vi "3.1-Make XY Graph.vi"() -> (0 "3.1-Midbrain Arbitrated Graph":T1)   [LabVIEW 2010]
uses:
  3.1-Midbrain Arbitrated Graph.ctl
  4-High Neurons/4.1-Midbrain Act Data.ctl
  3.0-Global.vi
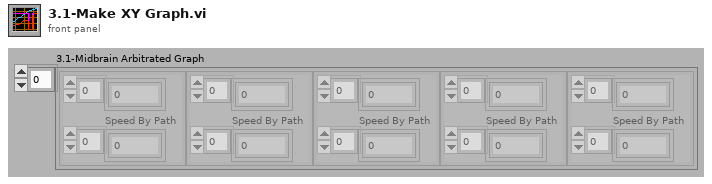
[diagram p1: front panel]
types:
  T1 = typedef "3.1-Midbrain Arbitrated Graph.ctl" = cluster{dbl[], "Speed By Path":dbl[]}[]
  T2 = enum16{"Set Joystick", "Read Joystick", "Set Forebrain", "Read Forebrain", "Set Limbic", "Read Limbic", "Set Cerebellum", "Read Cerebellum", "Set Arbitrated", "Read Arbitrated", "Set LIDAR", "Read LIDAR", "Read Shallow Map", "Set Shallow Map", "Read Decider", "Set Decider"}
  T3 = enum16{"Set Joystick", "Read Joystick", "Set Forebrain", "Read Forebrain", "Set Limbic", "Read Limbic", "Set Cerebellum", "Read Cerebellum", "Set Arbitrated", "Read Arbitrated", "Set LIDAR", "Read LIDAR", "Read Shallow Map", "Set Shallow Map"}
  T4 = enum16{"Set Midbrain Act Data", "Read Midbrain Act Data"}
  T5 = typedef "4.1-Midbrain Act Data.ctl" = cluster{"Arbitrated Array":sgl[], "Exploded Obstacles":sgl[], "Desired Change in Heading":sgl, "Desired Speed Fraction":sgl}
  T6 = enum16{"Steering Setpoints", "Desired Change in Heading"}
  T7 = enum16{"Set Joystick", "Read Joystick", "Set Forebrain", "Read Forebrain", "Set Limbic", "Read Limbic", "Set Cerebellum", "Read Cerebellum", "Set Arbitrated", "Read Arbitrated", "Set LIDAR", "Read LIDAR"}
  T8 = typedef "4.1.2-Act Neuron TD.ctl" = cluster{"Speed By Path":sgl[]}
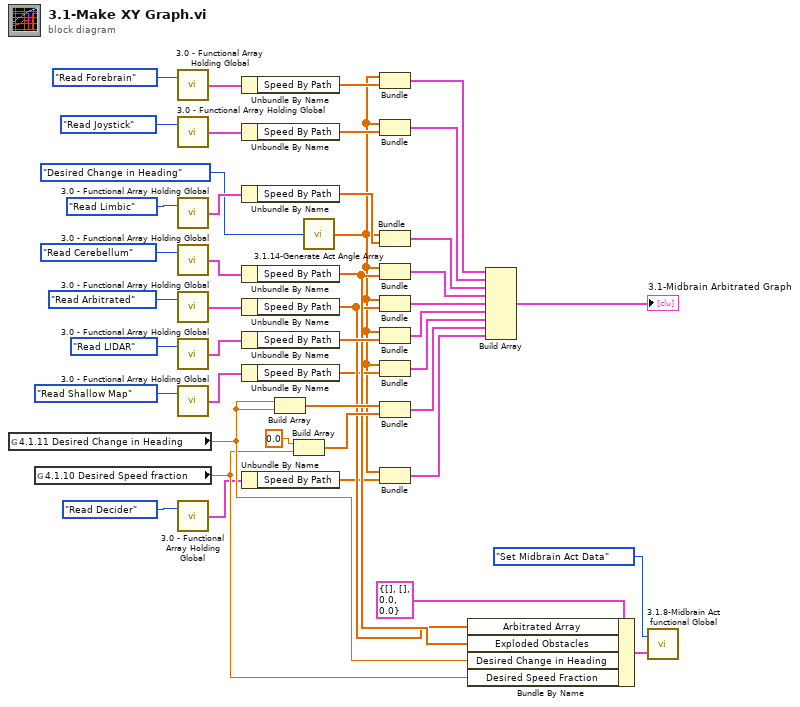
[diagram p0: block diagram]
diagram:
  n1 = global read "3.0-Global.vi" "4.1.11 Desired Change in Heading"() -> (w16:dbl)
  n2 = global read "3.0-Global.vi" "4.1.10 Desired Speed fraction"() -> (w11:dbl)
  n3 = call "3.0 - Functional Array Holding Global.vi"("Mode"=T7."Read Forebrain") -> ("Output Act Neurons"=w37:T8)  [unwired: 1 in]
  n4 = call "3.0 - Functional Array Holding Global.vi"("Mode"=T7."Read Joystick") -> ("Output Act Neurons"=w35:T8)  [unwired: 1 in]
  n5 = call "3.0 - Functional Array Holding Global.vi"("Mode"=T7."Read Limbic") -> ("Output Act Neurons"=w33:T8)  [unwired: 1 in]
  n6 = call "3.0 - Functional Array Holding Global.vi"("Mode"=T7."Read Cerebellum") -> ("Output Act Neurons"=w31:T8)  [unwired: 1 in]
  n7 = call "3.0 - Functional Array Holding Global.vi"("Mode"=T7."Read Arbitrated") -> ("Output Act Neurons"=w26:T8)  [unwired: 1 in]
  n8 = call "3.0 - Functional Array Holding Global.vi"("Mode"=T7."Read LIDAR") -> ("Output Act Neurons"=w29:T8)  [unwired: 1 in]
  n9 = call "3.0 - Functional Array Holding Global.vi"("Mode"=T3."Read Shallow Map") -> ("Output Act Neurons"=w9:T8)  [unwired: 1 in]
  n10 = call "3.0 - Functional Array Holding Global.vi"("Mode"=T2."Read Decider") -> ("Output Act Neurons"=w5:T8)  [unwired: 1 in]
  n11 = Unbundle By Name(w37) -> ("Speed By Path"=w39:sgl[])
  n12 = Unbundle By Name(w35) -> ("Speed By Path"=w42:sgl[])
  n13 = Unbundle By Name(w33) -> ("Speed By Path"=w44:sgl[])
  n14 = Unbundle By Name(w31) -> ("Speed By Path"=w15:sgl[])
  n15 = Unbundle By Name(w26) -> ("Speed By Path"=w14:sgl[])
  n16 = Unbundle By Name(w29) -> ("Speed By Path"=w28:sgl[])
  n17 = Unbundle By Name(w9) -> ("Speed By Path"=w8:sgl[])
  n18 = Unbundle By Name(w5) -> ("Speed By Path"=w3:sgl[])
  n19 = Build Array(w16, w16) -> (w23:dbl[])
  n20 = Build Array(0.0, w11) -> (w22:dbl[])
  n21 = call "3.1.14-Generate Act Angle Array.vi"("Enum"=T6."Desired Change in Heading") -> ("Array"=w2:dbl[])
  n22 = Bundle("Array"=w2, "Speed By Path"=w39) -> (w40:cluster{"Array":dbl[], "Speed By Path":sgl[]})  [unwired: 1 in]
  n23 = Bundle("Array"=w2, "Speed By Path"=w42) -> (w41:cluster{"Array":dbl[], "Speed By Path":sgl[]})  [unwired: 1 in]
  n24 = Bundle("Array"=w2, "Speed By Path"=w44) -> (w43:cluster{"Array":dbl[], "Speed By Path":sgl[]})  [unwired: 1 in]
  n25 = Bundle("Array"=w2, "Speed By Path"=w15) -> (w19:cluster{"Array":dbl[], "Speed By Path":sgl[]})  [unwired: 1 in]
  n26 = Bundle("Array"=w2, "Speed By Path"=w14) -> (w18:cluster{"Array":dbl[], "Speed By Path":sgl[]})  [unwired: 1 in]
  n27 = Bundle("Array"=w2, "Speed By Path"=w28) -> (w25:cluster{"Array":dbl[], "Speed By Path":sgl[]})  [unwired: 1 in]
  n28 = Bundle("Array"=w2, "Speed By Path"=w8) -> (w6:cluster{"Array":dbl[], "Speed By Path":sgl[]})  [unwired: 1 in]
  n29 = Bundle(w23, w22) -> (w7:cluster{dbl[], dbl[]})  [unwired: 1 in]
  n30 = Bundle("Array"=w2, "Speed By Path"=w3) -> (w1:cluster{"Array":dbl[], "Speed By Path":sgl[]})  [unwired: 1 in]
  n31 = Bundle By Name(cluster=T5 {"Arbitrated Array"=[], "Exploded Obstacles"=[], "Desired Change in Heading"=0.0, "Desired Speed Fraction"=0.0} ("4.1- Midbrain Act Data"), "Arbitrated Array"=w14, "Exploded Obstacles"=w15, "Desired Change in Heading"=w16, "Desired Speed Fraction"=w11) -> (w13:T5)
  n32 = Build Array(w40, w41, w43, w19, w18, w25, w6, w7, w1) -> (→"3.1-Midbrain Arbitrated Graph":cluster{"Array":dbl[], "Speed By Path":dbl[]}[])
  n33 = call "3.1.8-Midbrain Act functional Global.vi"("4.1- Midbrain Act Data"=w13, "Command"=T4."Set Midbrain Act Data") -> ()  [unwired: 1 out]
